vi "Checkbox Display.vi"(8 "[Checkboxes] Ref":refnum<vi>, 9 "Starting Row":i32, 10 "Checkbox Array":bool[](array[boolean]), 11 "Checkbox Refs":refnum<vi>[](array[refnum])) -> ()   [LabVIEW 2013]
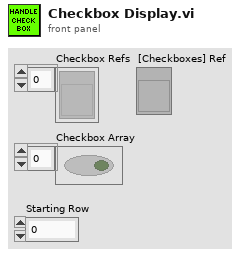
[diagram p1: front panel]
types:
  T1 = cluster{"[0]":bool, "[1]":bool, "[2]":bool, "[3]":bool, "[4]":bool, "[5]":bool, "[6]":bool, "[7]":bool, "[8]":bool, "[9]":bool, "[10]":bool, "[11]":bool}
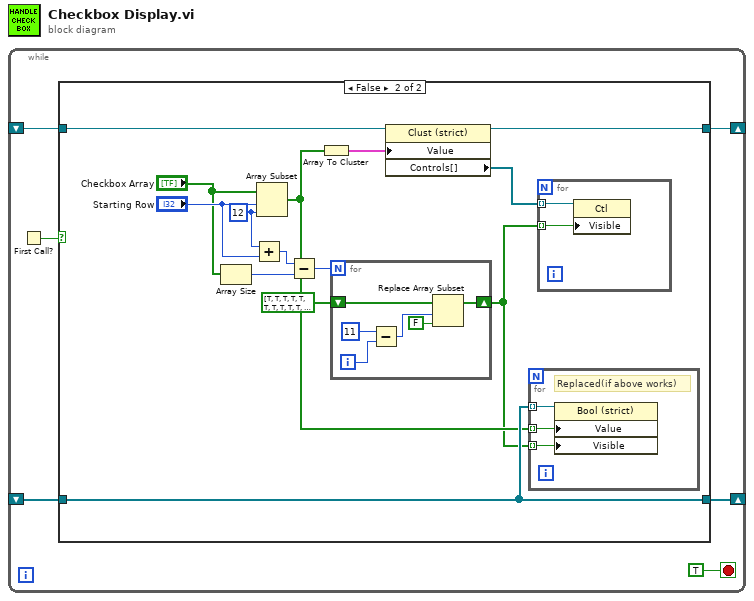
[diagram p0: block diagram]
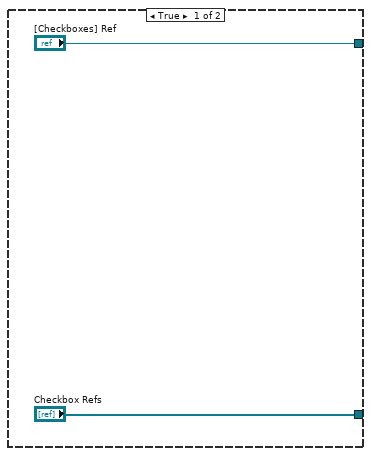
[diagram p2: hidden frame]
diagram:
  n1 = while {
    shift-right: [w3] -> _
    shift-left: _ -> [w4]
    shift-right: [w2] -> _
    shift-left: _ -> [w1]
    stop <- TRUE stop-if-true
    n2 = First Call?() -> (First Call?: T/F=w5:bool)
    n3 = case shown="False" w5 {
      tunnel: w4 -> [_ w16]
      tunnel: ["Checkbox Refs" w16] -> w3
      tunnel: ["[Checkboxes] Ref" w9] -> w2
      tunnel: w1 -> [_ w15]
      frame True {
      }
      frame False {
        w20 = 12 ("length")
        n4 = Array Size(array="Checkbox Array") -> (size(s)=w22:i32)
        n5 = Add(x=w20, y="Starting Row") -> (x+y=w21:i32)
        n6 = Array Subset(array="Checkbox Array", index="Starting Row", length=w20) -> (w12:bool[])
        n7 = Subtract(x=w21, y=w22) -> (x-y=w17:i32)
        n8 = Array To Cluster(array=w12) -> (cluster=w13:T1)
        n9 = for {
          N: w17 -> [_]
          shift-right: [w25] -> w10
          shift-left: bool[] [TRUE, TRUE, TRUE, TRUE, TRUE, TRUE, TRUE, TRUE, TRUE, TRUE, TRUE, TRUE] -> [w30]
          i -> [w29]
          n10 = Subtract(x=11, y=w29) -> (x-y=w27:i32)
          n11 = Replace Array Subset(array=w30, new element=FALSE ("new element/subarray"), index=w27) -> (w25:bool[])
        }
        n12 = property class="Clust (strict)"(reference=w15, "Value"=w13) -> (reference out=w9:refnum<vi>, "Controls[]"=w11:refnum<vi>[])  [unwired: 1 in, 1 out]
        n13 = for {
          tunnel: w12 -> [w33] mode=indexing
          tunnel: w16 -> [w32] mode=indexing
          tunnel: w10 -> [w31] mode=indexing
          # "Replaced(if above works)"
          n14 = property on="Property Node" class="Bool (strict)"(reference=w32, "Value"=w33, "Visible"=w31) -> ()  [unwired: 1 in, 2 out]
        }
        n15 = for {
          tunnel: w11 -> [w24] mode=indexing
          tunnel: w10 -> [w23] mode=indexing
          n16 = property class="Ctl"(reference=w24, "Visible"=w23) -> ()  [unwired: 1 in, 2 out]
        }
      }
    }
  }
